vi "Replace Call Chain Specifier.vi"(11 "format string":string) -> (3 "resulting string":string)   [LabVIEW 2018, in "Logging.lvlib" / "Format String.lvclass"]
uses:
  Format String.lvclass
  <vilib>/regexp/Match Regular Expression.xnode
panel:
  # "Connector Pane"
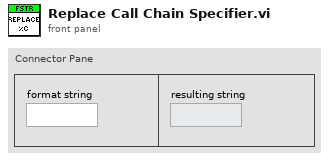
[diagram p1: front panel]
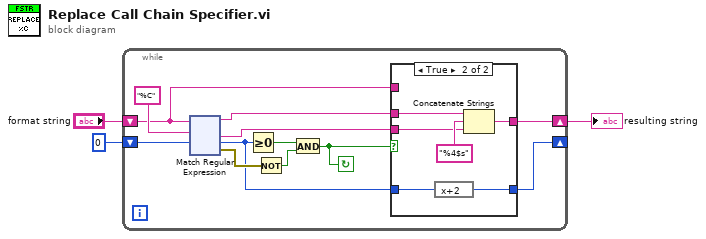
[diagram p0: block diagram]
diagram:
  n1 = while {
    shift-right: [w8] -> w2
    shift-left: "format string" -> [w9]
    shift-right: [w4] -> _
    shift-left: 0 ("offset (0)") -> [w6]
    stop <- w7 continue-if-true
    n2 = xnode "Match Regular Expression"("input string"=w9, "regular expression"="%C", "offset (0)"=w6) -> ("before match"=w11:string, "after match"=w10:string, "offset past match"=w5:i32, "error out"=w13:errorcluster)  [unwired: 3 in, 1 out]
    n3 = Greater Or Equal To 0?(x=w5) -> (x >= 0?=w14:bool)
    n4 = Not(x=w13) -> (.not. x?=w12:bool)
    n5 = And(x=w14, y=w12) -> (x .and. y?=w7:bool)
    n6 = case shown="True" w7 {
      tunnel: w11 -> [_ w140]
      tunnel: w10 -> [_ w138]
      tunnel: [w134 w137] -> w8
      tunnel: w9 -> [w134 _]
      tunnel: w5 -> [w133 w136]
      tunnel: [w133 w135] -> w4
      frame False {
      }
      frame True {
        n7 = expression code="x+2"(w136) -> (w135:i32)
        n8 = Concatenate Strings(w140, "%4$s" ("string"), w138) -> (w137:string)
      }
    }
  }
  "resulting string" <- w2
